vi "Core Actor - DISPLAY - Message (String).vi"(8 "error in (no error)":errorcluster, 9 "Value":string, 11 "Parent_Class in":refnum<class "Message_Distributor_Class.lvclass">) -> (0 "error out":errorcluster, 3 "Parent_Class out":refnum<class "Message_Distributor_Class.lvclass">)   [LabVIEW 2023, in "Actor_Message_Distributor.lvlib" / "Message_Distributor_Class.lvclass"]
uses:
  Message_Distributor_Class.lvclass
  Message_Distributor_Class.lvclass/Message_Distributor_Class.ctl
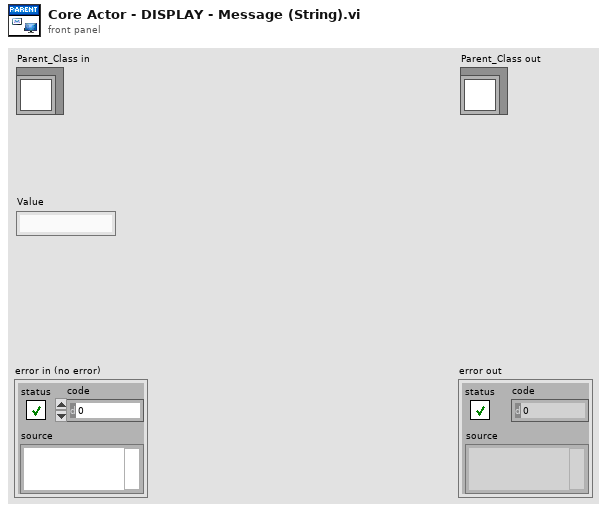
[diagram p1: front panel]
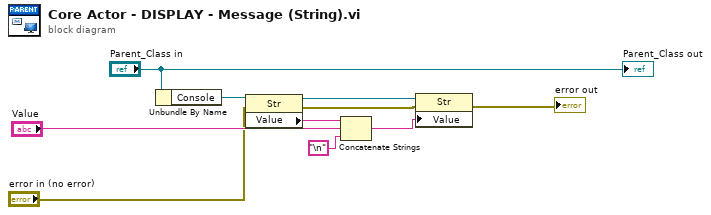
[diagram p0: block diagram]
diagram:
  n1 = Unbundle By Name("Parent_Class in") -> ("Console"=w9:refnum<vi>)
  n2 = property class="Str"(reference=w9, error in="error in (no error)") -> (reference out=w4:refnum<vi>, error out=w3:errorcluster, "Value"=w8:string)
  n3 = Concatenate Strings(w8, "Value", "\n") -> (w2:string)
  n4 = property class="Str"(reference=w4, error in=w3, "Value"=w2) -> (error out=→"error out":errorcluster)  [unwired: 1 out]
  "Parent_Class out" <- "Parent_Class in"
